vi "Update Color Pair Array.vi"(8 "error in (no error)":errorcluster, 9 "Color Pair Array":cluster{"Color":u32, "String":string}[](array[cluster]), 11 "3D Plot.lvclass in":refnum<class "3D Plot.lvclass">) -> (0 "error out":errorcluster, 3 "3D Plot.lvclass out":refnum<class "3D Plot.lvclass">)   [LabVIEW 2017, in "3D Plot.lvclass"]
uses:
  <vilib>/Math Plots/3D Math Plots/3D Plot/3D Plot/3D Plot.lvclass
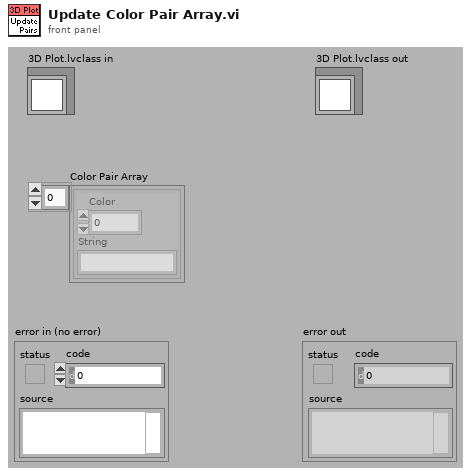
[diagram p1: front panel]
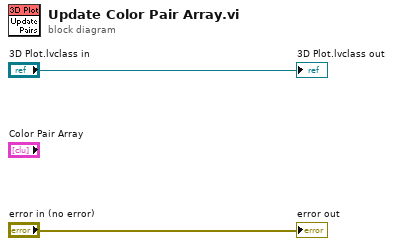
[diagram p0: block diagram]
diagram:
  "3D Plot.lvclass out" <- "3D Plot.lvclass in"
  "error out" <- "error in (no error)"
